vi "Initialise.vi"(8 "error in (no error)":errorcluster, 11 "Sink in":refnum<class "Sink.lvclass">) -> (0 "error out":errorcluster, 3 "Sink out":refnum<class "Sink.lvclass">)   [LabVIEW 2020, in "LV Log.lvlib" / "Sink.lvclass"]
uses:
  Sink.lvclass
  Sink.lvclass/Sink.ctl
  <vilib>/ErrorRing/Error Ring.xnode
  <vilib>/Utility/error.llb/Error Cluster From Error Code.vi
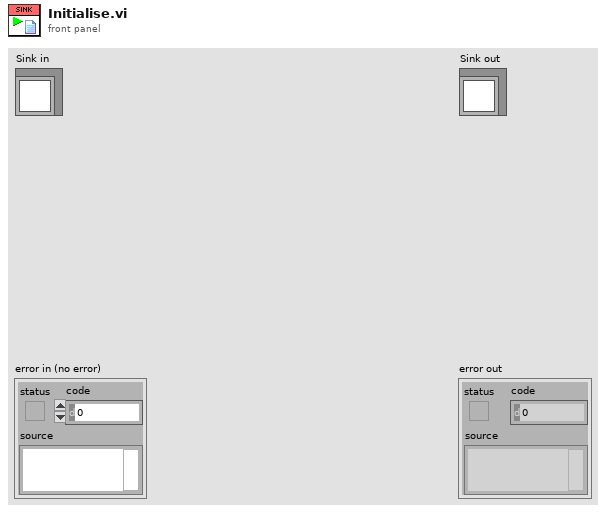
[diagram p1: front panel]
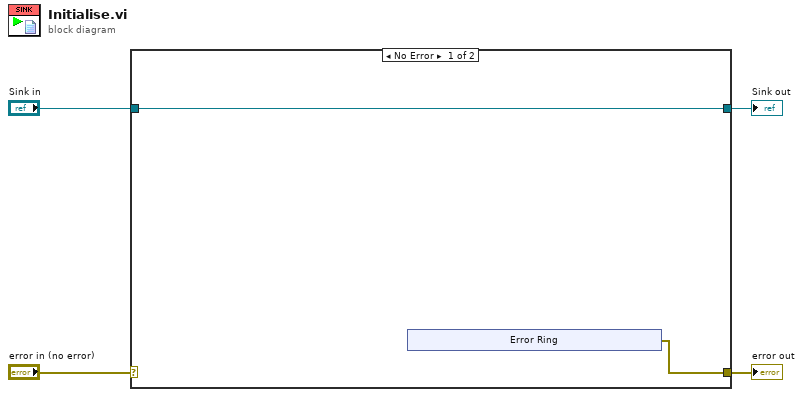
[diagram p0: block diagram]
diagram:
  n1 = case shown="No Error" "error in (no error)" {
    selector: "error in (no error)" -> [_ w13]
    tunnel: [w5 w13] -> w3
    tunnel: [w6 w12] -> w1
    tunnel: "Sink in" -> [w6 w12]
    frame No Error {
      n2 = xnode "Error Ring"() -> ("error out"=w5:errorcluster)
    }
    frame Error {
    }
  }
  "error out" <- w3
  "Sink out" <- w1
